vi "telToClient.vi"(8 "error in (no error)":errorcluster, 9 "queueOptions":T1={"EnqueueOptions"=enum."normal enqueue", "Timeout"=0}, 10 "Telemetry":T3, 11 "TcpServerTel in":refnum<class "TcpServerTel.lvclass">) -> (0 "error out":errorcluster, 3 "TcpServerTel out":refnum<class "TcpServerTel.lvclass">)   [LabVIEW 2018, in "TcpServerTel.lvclass"]
doc: "Send the telemetry to the TCP Client."
uses:
  TcpServerTel.lvclass
  home/pcortes/github/ts_labview_tcp_json/src/TcpServerBase/TcpServerBase.lvclass
  typedef/telTypeDef.ctl
  typedef/queueOptionsTypeDef.ctl
  typedef/enqueueOptionsTypeDef.ctl
  TcpServerBase/typedef/msgTypeDef.ctl
  TcpServerBase/TcpServerBase.lvclass
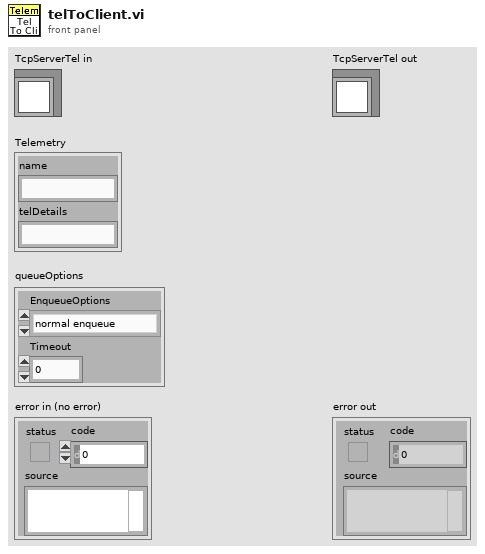
[diagram p1: front panel]
types:
  T1 = typedef "TcpServerTel.lvclass/queueOptionsTypeDef.ctl" = cluster{"EnqueueOptions":T2, "Timeout":i32}
  T2 = typedef "TcpServerTel.lvclass/enqueueOptionsTypeDef.ctl" = enum16{"lossy enqueue", "normal enqueue"}
  T3 = typedef "TcpServerTel.lvclass/telTypeDef.ctl" = cluster{"name":string, "telDetails":string}
  T4 = typedef "TcpServerBase.lvclass/msgTypeDef.ctl" = cluster{"msgName":string, "msgDetails":string}
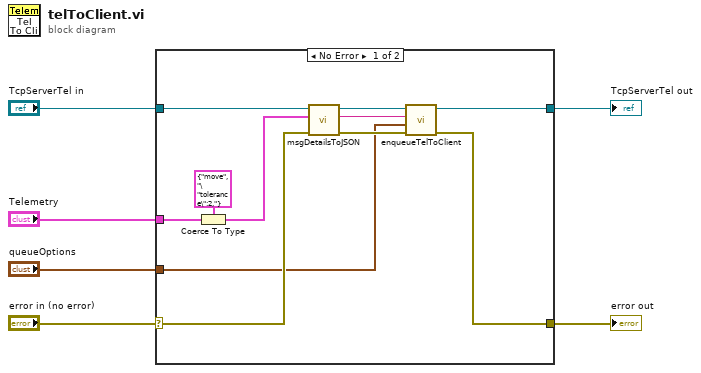
[diagram p0: block diagram]
diagram:
  n1 = case shown="No Error" "error in (no error)" {
    selector: "error in (no error)" -> [w14 w19]
    tunnel: [w13 w19] -> w5
    tunnel: [w7 w18] -> w1
    tunnel: "TcpServerTel in" -> [w15 w18]
    tunnel: "Telemetry" -> [w12 _]
    tunnel: "queueOptions" -> [w9 _]
    frame No Error {
      n2 = Coerce To Type(0:w12, 1:T4 {"msgName"="move", "msgDetails"="\"tolerance\":2,"} ("msgData")) -> (2:w11:T4)
      n3 = call "msgDetailsToJSON.vi"("error in (no error)"=w14, "msgData"=w11, "TcpServerBase in"=w15) -> ("error out"=w17:errorcluster, "JSON string"=w16:string, "TcpServerBase out"=w8:refnum<class "TcpServerTel.lvclass">)  [unwired: 6 in]
      n4 = call "enqueueTelToClient.vi"("error in (no error)"=w17, "queueOptions"=w9, "elements to enqueue"=w16, "TcpServerTel in"=w8) -> ("error out"=w13:errorcluster, "TcpServerTel out"=w7:refnum<class "TcpServerTel.lvclass">)  [unwired: 6 in]
    }
    frame Error {
    }
  }
  "error out" <- w5
  "TcpServerTel out" <- w1
